vi "gfitsio-read-key-string.vi"(7 "keyname":string, 8 "error in (no error)":errorcluster, 9 "default value":string, 11 "gfits refnum":T1) -> (0 "error out":errorcluster, 1 "comment":string, 2 "value":string, 3 "dup gfits refnum":T1)   [LabVIEW 2019, in "gfitsio.lvlib"]
doc: "Return the specified keyword. <B>default value</B> specifies the desired returned data type of the keyword value. Data type conversion will be performed for numeric values if the keyword value does not have the same data type. If the keyword does not exist or an error occurs <B>value</B> will be equal to <B>default value</B>."
uses:
  gfitsio.lvlib
  gfitsio-refnum.ctl
  cfitsio-datatypes.ctl
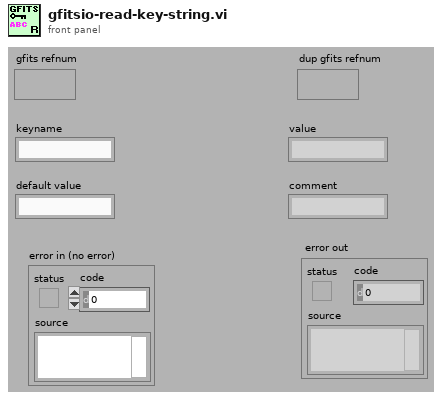
[diagram p1: front panel]
types:
  T1 = typedef "gfitsio.lvlib/gfitsio-refnum.ctl" = refnum<k1>
  T2 = typedef "gfitsio.lvlib/cfitsio-datatypes.ctl" = i32
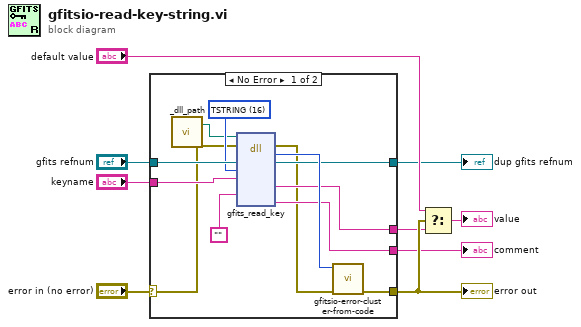
[diagram p0: block diagram]
diagram:
  n1 = case shown="No Error" "error in (no error)" {
    selector: "error in (no error)" -> [w12 w23]
    tunnel: [w20 w23] -> w4
    tunnel: "gfits refnum" -> [w18 w22]
    tunnel: [w19 w22] -> w1
    tunnel: "keyname" -> [w16 _]
    tunnel: [w15 _] -> w2
    tunnel: [w14 _] -> w3
    frame No Error {
      w17 = T2 16 items=["TBIT"=1, "TBYTE  (U8)"=11, "TSBYTE  (I8)"=12, "TLOGICAL"=14, "TSTRING"=16, "TUSHORT  (U16)"=20, "TSHORT  (I16)"=21, "TUINT"=31, "TULONG  (U32)"=40, "TLONG  (I32)"=41, "TFLOAT  (SGL)"=42, "TLONGLONG  (I64)"=81, "TDOUBLE"=82, "TCOMPLEX  (CSG)"=83, "TDOUBLECOMPLEX  (CDB)"=163] ("cfitsio datatype")
      n2 = call "_dll_path.vi"() -> ("Path"=w10:path)  [unwired: 1 in]
      n3 = dll-call lib="?" fn="gfits_read_key"(path in=w10, error in=w12, "refnum"=w18, "datatype"=w17, "keyname"=w16, "units"="") -> (error out=w11:errorcluster, "return type"=w21:i32, "refnum"=w19:T1, "value"=w15:string, "comment"=w14:string)  [unwired: 3 in, 4 out]
      n4 = call "gfitsio-error-cluster-from-code.vi"("error in (no error)"=w11, "error code"=w21) -> ("error out"=w20:errorcluster)  [unwired: 9 out]
    }
    frame Error {
    }
  }
  "error out" <- w4
  "dup gfits refnum" <- w1
  "comment" <- w3
  n5 = Select(t="default value", s=w4, f=w2) -> (s? t:f=→"value":string)
